vi "NT Client.vi"(4 "Update Time":i32=100, 5 "Cancel Ref":refnum<notifier>, 6 "Tracing":bool, 7 "Automatic restart":bool=TRUE, 8 "user event ref":refnum<user-event>, 9 "Client Name":string, 10 "timeout ms (1000)":i32=1000, 11 "Server IP Address":string="localhost") -> ()   [LabVIEW 2017]
doc: "Place this VI in the Dashboard or other client applications so that it can run in parallel with the other tasks. Provide the robot IP address so that it can know where to find the server.\n\nYou normally want the restart option to be true, but if you have your own restart strategy, you can disable it. Tracing is useful when debugging. Similarly, the disconnect timout may need to be raised if setting breakpoints. The user event ref will publish the client activities so that other elements of the dashboard are notified when packets are processed."
uses:
  <vilib>/Rock Robotics/Network Tables/NT Event Type.ctl
  <vilib>/Rock Robotics/Network Tables/Protocol Operations.ctl
  <vilib>/Rock Robotics/Network Tables/Field Data.ctl
  <vilib>/Rock Robotics/Network Tables/Field Type.ctl
  <vilib>/Rock Robotics/Network Tables/Sequence.ctl
  <vilib>/Rock Robotics/Network Tables/NT Globals.vi
panel:
  in  "Cancel":bool=TRUE
  out "Trace Strings":string
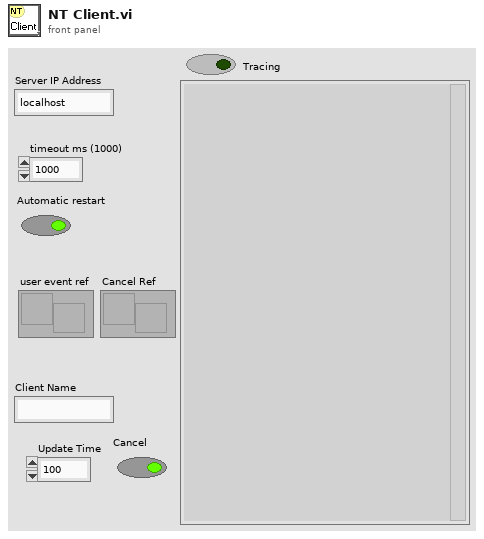
[diagram p1: front panel]
types:
  T1 = enum16{"Add Cnx", "Remove Cnx", "Retrieve List", "Cnx Inited"}
  T2 = typedef "NT Event Type.ctl" = cluster{"Operation":T3, "Name":string, "Field Value":T4}
  T3 = typedef "Protocol Operations.ctl" = enum16{"Unknown", "Keep Alive", "Client Hello", "Version not supported", "Server Hello Complete", "Assign", "Update", "No Op", "Server Hello", "Client Hello Complete", "Update Flags", "Delete Entry", "Delete All", "RPC Exec", "RPC Response"}
  T4 = typedef "Field Data.ctl" = cluster{"Dbl":dbl, "String":string, "Type":T5, "Boolean":bool, "Sequence #":T6, "Flags":u8}
  T5 = typedef "Field Type.ctl" = enum8{"Invalid", "Bool", "Numeric", "String", "Raw", "Boolean Array", "Numeric Array", "String Array", "RPC"}
  T6 = typedef "Sequence.ctl" = u16
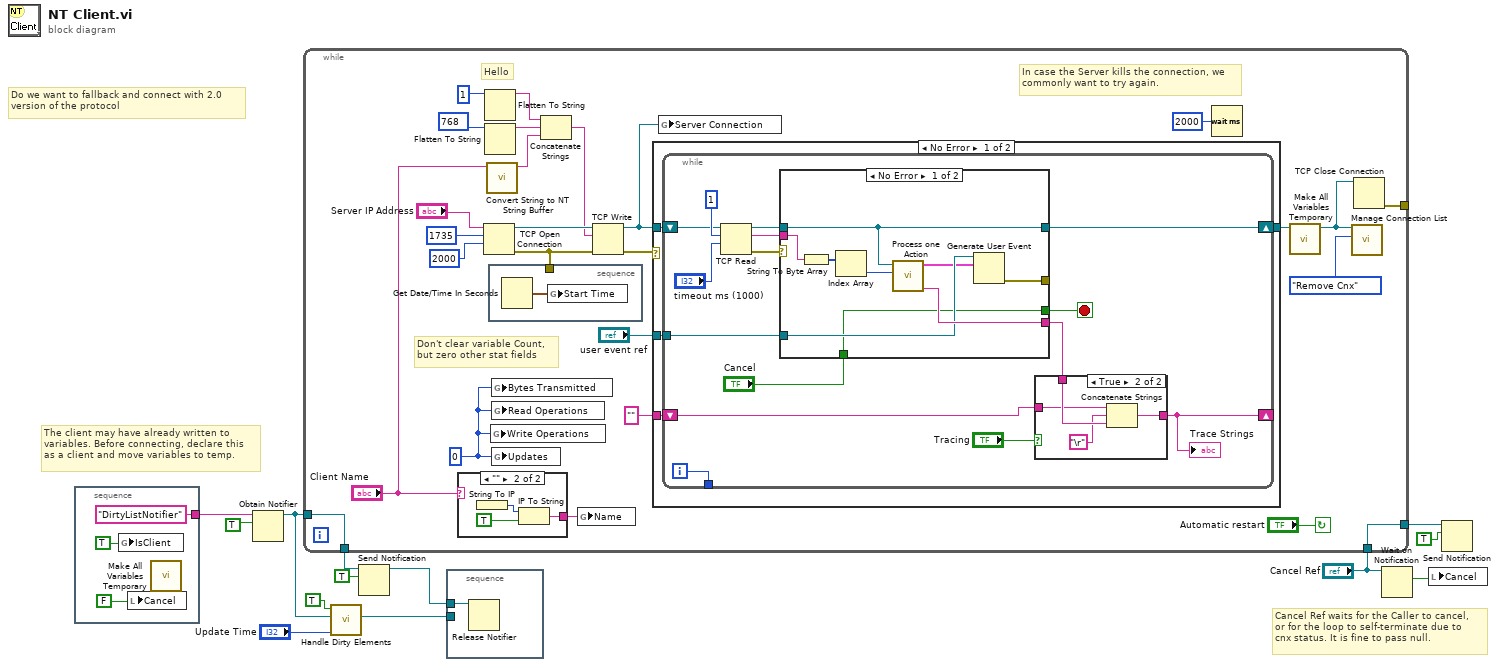
[diagram p0: block diagram]
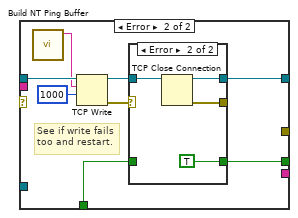
[diagram p3: hidden frame]
diagram:
  # "Do we want to fallback and connect with 2.0\nversion of the protocol"
  # "Cancel Ref waits for the Caller to cancel,\nor for the loop to self-terminate due to\ncnx status. It is fine to pass null."
  # "The client may have already written to\nvariables. Before connecting, declare this\nas a client and move variables to temp."
  n1 = stacked-sequence {
    tunnel: ["DirtyListNotifier" ("name (unnamed)")] -> w6
    frame #0 {
      n2 = global write "NT Globals.vi" "IsClient"(TRUE ("IsClient")) -> ()
      n3 = local write "Cancel"(FALSE ("IsClient")) -> ()
      n4 = call <vilib>:"Make All Variables Temporary.vi"() -> ()  [unwired: 11 in, 1 out]
    }
  }
  n5 = Obtain Notifier(name (unnamed)=w6, notification data type=TRUE ("IsClient")) -> (notifier out=w10:refnum<notifier>)  [unwired: 2 in, 2 out]
  n6 = while {
    tunnel: [w37] -> _
    tunnel: w10 -> [w21]
    tunnel: [w21] -> w11
    tunnel: [w20] -> w2
    tunnel: "Cancel Ref" -> [w20]
    stop <- "Automatic restart" continue-if-true
    w23 = 0 ("Updates")
    # "Don't clear variable Count,\nbut zero other stat fields"
    # "Hello"
    # "In case the Server kills the connection, we\ncommonly want to try again."
    n7 = case shown="\"\"" "Client Name" {
      selector: "Client Name" -> [w92 _]
      tunnel: [w92 w93] -> w24
      frame Default {
      }
      frame "" {
        n8 = String To IP() -> (0:w95:u32)  [unwired: 1 in]
        n9 = IP To String(1:TRUE ("dot notation? (F)"), 2:w95) -> (0:w93:string)
      }
    }
    n10 = TCP Open Connection(address="Server IP Address", remote port or service name=u16 1735 ("port"), timeout ms (60000)=2000) -> (connection ID=w36:refnum<k5>, error out=w25:errorcluster)  [unwired: 2 in]
    n11 = Flatten To String(anything=u8 1) -> (data string=w32:string)  [unwired: 3 in, 2 out]
    n12 = Flatten To String(anything=u16 768) -> (data string=w31:string)  [unwired: 3 in, 2 out]
    n13 = call <vilib>:"Convert String to NT String Buffer.vi"("LV Buffer"="Client Name") -> ("NT Buffer"=w18:string)  [unwired: 10 in]
    n14 = stacked-sequence {
      tunnel: w25 -> [_]
      frame #0 {
        n15 = Get Date/Time In Seconds() -> (seconds since 1Jan1904=w96:timestamp)
        n16 = global write "NT Globals.vi" "Start Time"(w96) -> ()
      }
    }
    n17 = global write "NT Globals.vi" "Write Operations"(w23) -> ()
    n18 = global write "NT Globals.vi" "Bytes Transmitted"(w23) -> ()
    n19 = global write "NT Globals.vi" "Read Operations"(w23) -> ()
    n20 = global write "NT Globals.vi" "Updates"(w23) -> ()
    n21 = Concatenate Strings(w32, w31, w18) -> (w30:string)
    n22 = global write "NT Globals.vi" "Name"(w24) -> ()
    n23 = TCP Write(connection ID=w36, data in=w30, error in (no error)=w25) -> (connection ID out=w35:refnum<k5>, error out=w22:errorcluster)  [unwired: 1 in, 1 out]
    n24 = case shown="No Error" w22 {
      tunnel: "" -> [w46 _]
      tunnel: w35 -> [w45 w91]
      tunnel: "user event ref" -> [w44 _]
      tunnel: [w43 w91] -> w27
      frame No Error {
        n25 = while {
          shift-right: [w57] -> w43
          shift-left: w45 -> [w59]
          tunnel: [w53] -> _
          shift-right: [w50] -> _
          shift-left: w46 -> [w51]
          tunnel: w44 -> [w48]
          i -> [w53]
          stop <- w56 stop-if-true
          n26 = TCP Read(connection ID=w59, bytes to read=1 ("timeout ms (25000)"), 9:"timeout ms (1000)") -> (connection ID out=w58:refnum<k5>, data out=w55:string, error out=w54:errorcluster)  [unwired: 2 in]
          n27 = case shown="No Error" w54 {
            tunnel: w55 -> [w75 _]
            tunnel: [w73 w83] -> w57
            tunnel: w58 -> [w73 w82]
            tunnel: [w67 w78] -> w56
            tunnel: [w71 _] -> w52
            tunnel: w48 -> [w70 _]
            tunnel: [w68 _] -> _
            tunnel: "Cancel" -> [w67 w76]
            frame No Error {
              n28 = String To Byte Array(string=w75) -> (unsigned byte array=w74:u8[])
              n29 = Index Array(array=w74) -> (element=w72:u8)  [unwired: 1 in]
              n30 = call <vilib>:"Process one Action.vi"("First Byte"=w72, "connection ID"=w73) -> ("Debug Sring"=w71:string, "NT Event Data"=w69:T2)  [unwired: 8 in]
              n31 = Generate User Event(user event=w70, event data cluster=w69) -> (error out=w68:errorcluster)  [unwired: 2 in, 1 out]
            }
            frame Error {
              # "See if write fails\ntoo and restart."
              n32 = call <vilib>:"Build NT Ping Buffer.vi"() -> ("Data Buffer"=w77:string)  [unwired: 11 in]
              n33 = TCP Write(connection ID=w82, data in=w77, 9:1000 ("timeout ms (25000)")) -> (connection ID out=w81:refnum<k5>, error out=w79:errorcluster)  [unwired: 1 in, 1 out]
              n34 = case shown="Error" w79 {
                selector: w79 -> [w85 _]
                tunnel: [w86 w90] -> w83
                tunnel: [w85 w89] -> _
                tunnel: w81 -> [w86 w88]
                tunnel: [w84 TRUE] -> w78
                tunnel: w76 -> [w84 _]
                frame No Error {
                }
                frame Error {
                  n35 = TCP Close Connection(connection ID=w88) -> (connection ID out=w90:refnum<k5>, error out=w89:errorcluster)  [unwired: 2 in]
                }
              }
            }
          }
          n36 = case shown="True" "Tracing" {
            tunnel: w52 -> [w62 w66]
            tunnel: w51 -> [_ w65]
            tunnel: [w62 w63] -> w50
            frame False {
            }
            frame True {
              n37 = Concatenate Strings(w65, "\r", w66) -> (w63:string)
            }
          }
          "Trace Strings" <- w50
        }
      }
      frame Error {
      }
    }
    n38 = global write "NT Globals.vi" "Server Connection"(w35) -> ()
    n39 = Wait (ms)(milliseconds to wait=u32 2000) -> ()  [unwired: 1 out]
    n40 = call <vilib>:"Make All Variables Temporary.vi"("connection ID"=w27) -> ("connection ID 2"=w26:refnum<k5>)  [unwired: 10 in]
    n41 = call <vilib>:"Manage Connection List.vi"("Operation"=T1."Remove Cnx", "connection ID"=w26) -> ()  [unwired: 7 in, 3 out]
    n42 = TCP Close Connection(connection ID=w26) -> (error out=w37:errorcluster)  [unwired: 2 in, 1 out]
  }
  n43 = call <vilib>:"Handle Dirty Elements.vi"("Update Time"="Update Time", "notifier out"=w10, "IsClient"=TRUE) -> ("notifier out 2"=w7:refnum<notifier>)  [unwired: 8 in]
  n44 = Send Notification(notification=TRUE, notifier=w11) -> (notifier out=w8:refnum<notifier>)  [unwired: 1 in, 1 out]
  n45 = stacked-sequence {
    tunnel: w8 -> [w97]
    tunnel: w7 -> [_]
    frame #0 {
      n46 = Release Notifier(notifier=w97) -> ()  [unwired: 2 in, 3 out]
    }
  }
  n47 = Wait on Notification(notifier="Cancel Ref") -> (notification=w4:bool)  [unwired: 3 in, 3 out]
  n48 = local write "Cancel"(w4) -> ()
  n49 = Send Notification(notification=TRUE, notifier=w2) -> ()  [unwired: 1 in, 2 out]
